vi "DWDT Digital Size.vi"(8 "error in (no error)":errorcluster, 11 "digital waveform in":digitalwaveform(waveform)={"t0"=timestamp(0 s since 1904-01-01), "dt"=0.0, "Y"={"transitions"=[], "data"=[]}, "error"={"status"=FALSE, "code"=37421928, "source"=""}}) -> (0 "error out":errorcluster, 1 "number of signals":i32, 2 "number of samples":i32, 3 "digital waveform out":digitalwaveform(waveform)={"t0"=timestamp(0 s since 1904-01-01), "dt"=0.0, "Y"={"transitions"=[], "data"=[]}, "error"={"status"=FALSE, "code"=37421928, "source"=""}})   [LabVIEW 2020]
doc: "Returns the number of samples and signals contained in the digital input. Wire data to the <B>digital waveform in</B> input to determine the polymorphic instance to use or manually select the instance."
panel:
  in  "Empty Digital Waveform":digitalwaveform(waveform)={"t0"=timestamp(0 s since 1904-01-01), "dt"=0.0, "Y"={"transitions"=[], "data"=[]}, "error"={"status"=FALSE, "code"=37421928, "source"=""}}
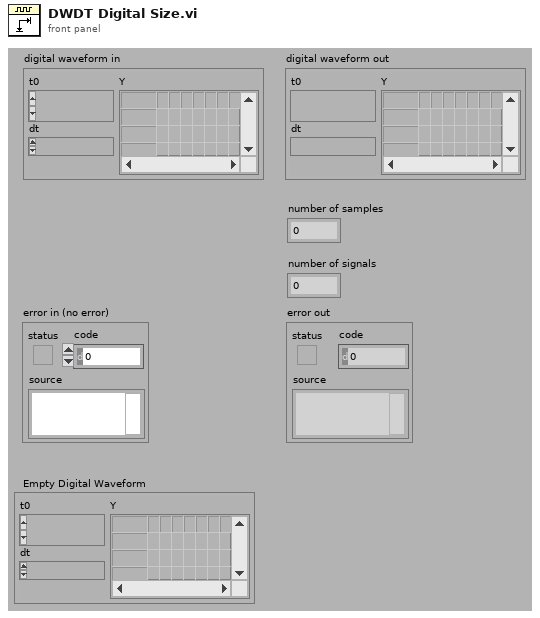
[diagram p1: front panel]
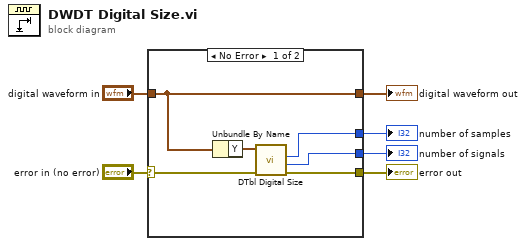
[diagram p0: block diagram]
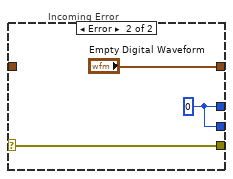
[diagram p2: hidden frame]
diagram:
  n1 = case shown="No Error" "error in (no error)" {
    selector: "error in (no error)" -> [w10 w15]
    tunnel: "digital waveform in" -> [w8 _]
    tunnel: [w8 "Empty Digital Waveform"] -> w5
    tunnel: [w11 w14] -> w6
    tunnel: [w9 w15] -> w3
    tunnel: [w12 w14] -> w1
    frame No Error {
      n2 = Unbundle By Name(w8) -> ("Y"=w7:digitaldata)
      n3 = call "DTbl Digital Size.vi"("error in (no error)"=w10, "digital data in"=w7) -> ("error out"=w9:errorcluster, "number of signals"=w11:i32, "number of samples"=w12:i32)  [unwired: 6 in, 1 out]
    }
    frame Error {
      w14 = 0
      # "Incoming Error"
    }
  }
  "number of signals" <- w6
  "digital waveform out" <- w5
  "error out" <- w3
  "number of samples" <- w1
